vi "Resonance Analyzer.vi"() -> ()   [LabVIEW 2015]
uses:
  <vilib>/imath/engines/lvmath2/RunTimeEngine/Managers/WorkSpace/UID Generator.vi
  <vilib>/imath/engines/lvmath2/RunTimeEngine/BuiltInFunctions/linramp/NIMS_linramp.vi
  <vilib>/imath/engines/lvmath2/RunTimeEngine/RunTimeType/NIMS_RunTimeType_From StrictType (excl LVString).vi
  <instcachedir>/0/NIMS_RunTimeType_From StrictType (excl LVString)_EB1C38A9BC5048DA9ABDA8F781E54D21.lvgen/NIMS_RunTimeType_From StrictType (excl LVString)_EB1C38A9BC5048DA9ABDA8F781E54D21_000.vi
  <vilib>/imath/engines/lvmath2/RunTimeEngine/LocalVariableDefStatement/MC_LocalVariableDefStatement_Display.vi
  <vilib>/imath/engines/lvmath2/RunTimeEngine/ArithmeticOperatorToken/NIMS_ArithmeticOperator_rightdivmx.vi
  <instcachedir>/0/NIMS_ArithmeticOperator_rightdivmx_C61A2D056ED24171800131CCD8A24414.lvgen/NIMS_ArithmeticOperator_rightdivmx_C61A2D056ED24171800131CCD8A24414_000.vi
  <vilib>/imath/engines/lvmath2/RunTimeEngine/ArithmeticOperatorToken/NIMS_ArithmeticOperator_minus.vi
  <instcachedir>/0/NIMS_ArithmeticOperator_minus_8228ED1EA52B4CB8A68367813E4B0C9D.lvgen/NIMS_ArithmeticOperator_minus_8228ED1EA52B4CB8A68367813E4B0C9D_002.vi
  <vilib>/imath/engines/lvmath2/RunTimeEngine/ArithmeticOperatorToken/NIMS_ArithmeticOperator_powermx(M,M).vi
  <vilib>/imath/engines/lvmath2/RunTimeEngine/ArithmeticOperatorToken/NIMS_ArithmeticOperator_rightdivmx(C,C).vi
  <instcachedir>/0/NIMS_ArithmeticOperator_rightdivmx(C,C)_8AB7F1F477EE4166BF59ADE0F95BCF66.lvgen/NIMS_ArithmeticOperator_rightdivmx(C,C)_8AB7F1F477EE4166BF59ADE0F95BCF66_000.vi
  <vilib>/imath/engines/lvmath2/RunTimeEngine/ErrorHandling/NIMS_Create Error From Enums.vi
  <vilib>/imathl/engines/lvmath/Functions/Error Handling/Create Error.vi
  <vilib>/imath/engines/lvmath2/RunTimeEngine/Managers/SymbolTable/Clear UID.vi
  <vilib>/imath/engines/lvmath2/RunTimeEngine/NodeEndStatement/NIMS_NodeEndStatement_Output.vi
  <instcachedir>/0/NIMS_NodeEndStatement_Output_53EC0D466D134D7ABD903AC30B43404B.lvgen/NIMS_NodeEndStatement_Output_53EC0D466D134D7ABD903AC30B43404B_005.vi
  <vilib>/imath/engines/lvmath2/RunTimeEngine/ErrorHandling/NIMS_Finalize Error.vi
  <vilib>/Utility/file.llb/Read Delimited Spreadsheet (DBL).vi
  <vilib>/imath/engines/lvmath2/RunTimeEngine/Managers/SymbolTable/NIMS_WorkSpace.lvlib
panel:
  out "best fit":dynamicdata(graph)
  in  "Tab Control":enum32{"Simulation", "Experiment"}(tab)
  in  "Cluster":T1
  out "Cluster 2":T2
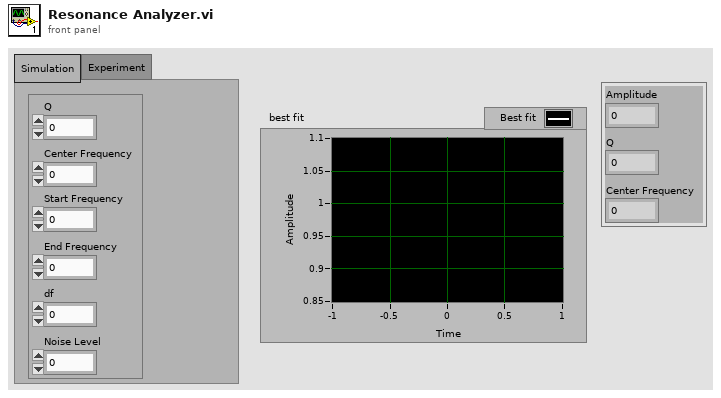
[diagram p1: front panel]
types:
  T1 = cluster{"Q":dbl, "Center Frequency":dbl, "Start Frequency":dbl, "End Frequency":dbl, "df":dbl, "Noise Level":dbl}
  T2 = cluster{"Amplitude":dbl, "Q":dbl, "Center Frequency":dbl}
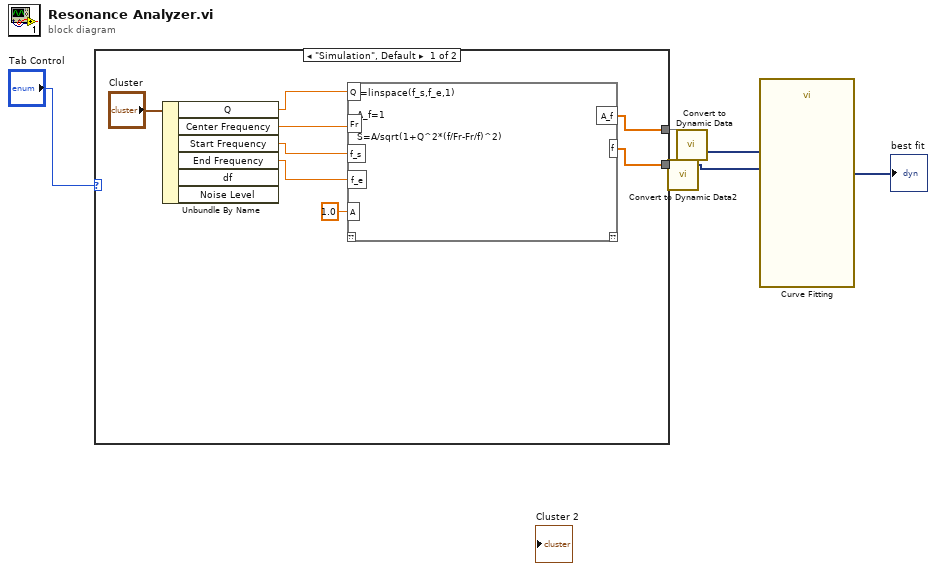
[diagram p0: block diagram]
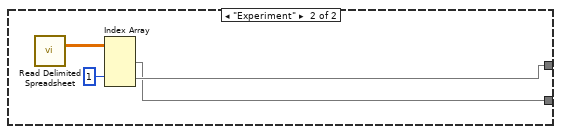
[diagram p2: hidden frame]
diagram:
  n1 = case shown="\"Simulation\", Default" "Tab Control" {
    tunnel: [w7 w151] -> w4
    tunnel: [w8 w150] -> w1
    frame "Simulation", Default {
      n2 = Unbundle By Name("Cluster") -> ("Q"=w13:dbl, "Center Frequency"=w12:dbl, "Start Frequency"=w11:dbl, "End Frequency"=w10:dbl)  [unwired: 2 out]
      n3 = mathscript code="f=linspace(f_s,f_e,1)\n\nA_f=1\n\nS=A/sqrt(1+Q^2*(f/Fr-Fr/f)^2)"("f_s"=w11, "Fr"=w12, "A"=1.0, "Q"=w13, "f_e"=w10) -> ("A_f"=w7:dbl[], "f"=w8:dbl[])  [unwired: 1 in, 1 out]
    }
    frame "Experiment" {
      n4 = call-poly <vilib>:"Read Delimited Spreadsheet.vi"() -> ("all rows"=w152:dbl[][])  [unwired: 10 in, 5 out]
      n5 = Index Array(array=w152, index (row) #2=1 ("index (row)")) -> (element #1=w150:dbl[], element #2=w151:dbl[])  [unwired: 3 in]
    }
  }
  n6 = call "Convert to Dynamic Data2"("Array"=w1) -> ("Dynamic Data Type"=w2:dynamicdata)  [unwired: 3 in]
  n7 = call "Convert to Dynamic Data"("Array"=w4) -> ("Dynamic Data Type"=w3:dynamicdata)  [unwired: 3 in]
  n8 = call "Curve Fitting"("Locations"=w2, "Signals"=w3) -> ("best fit"=→"best fit":dynamicdata)  [unwired: 5 in, 4 out]
